vi "Update Status on Result.vi"(8 "error in (no error)":errorcluster, 10 "Result":T1, 11 "Execution UI V2 in":refnum<class "Execution UI V2.lvclass">) -> (0 "error out":errorcluster, 3 "Execution UI V2 out":refnum<class "Execution UI V2.lvclass">)   [LabVIEW 2020, in "Execution UI V2.lvclass"]
uses:
  Execution UI V2.lvclass
  Result/Result.ctl
  Result/Status.ctl
  Result/Type.ctl
  Result/Result.lvlib
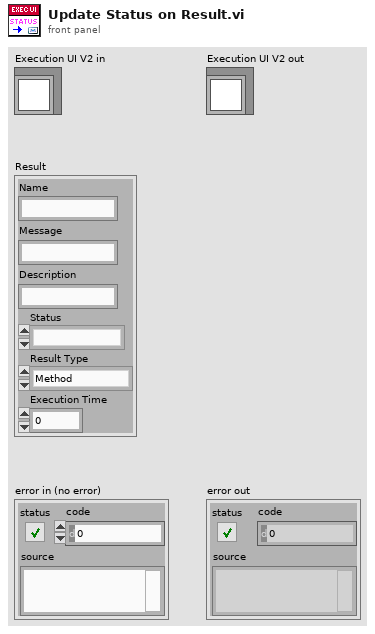
[diagram p1: front panel]
types:
  T1 = typedef "Result.lvlib/Result.ctl" = cluster{"Name":string, "Message":string, "Description":string, "Status":T2, "Result Type":T3, "Execution Time":dbl}
  T2 = typedef "Result.lvlib/Status.ctl" = enum16{"", "Passed", "Failed", "Error", "Skipped", "Setup Error", "Broken", "Teardown Error"}
  T3 = typedef "Result.lvlib/Type.ctl" = enum16{"Method", "Case", "Suite", "Pass", "Fail", "Skip", "Pass if", "Fail if", "Pass if Error", "Fail if Error", "Pass if Equal", "Fail if Equal"}
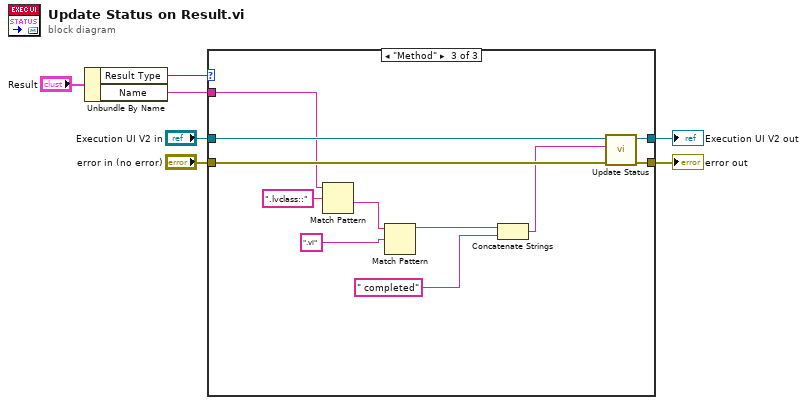
[diagram p0: block diagram]
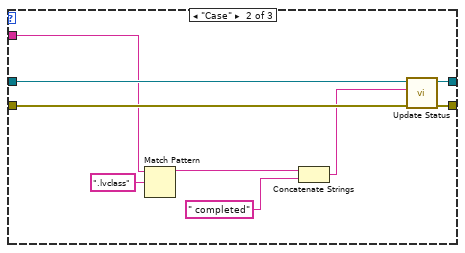
[diagram p3: hidden frame]
diagram:
  n1 = Unbundle By Name("Result") -> ("Result Type"=w7:T3, "Name"=w1:string)
  n2 = case shown="\"Method\"" w7 {
    tunnel: "Execution UI V2 in" -> [w9 w18 w29]
    tunnel: [w9 w17 w28] -> w3
    tunnel: "error in (no error)" -> [w8 w16 w27]
    tunnel: [w8 w15 w26] -> w5
    tunnel: w1 -> [_ w13 w21]
    frame Default {
    }
    frame "Case" {
      n3 = Match Pattern(string=w13, regular expression=".lvclass") -> (before substring=w11:string)  [unwired: 1 in, 3 out]
      n4 = Concatenate Strings(w11, " completed" ("Status")) -> (w10:string)
      n5 = call "Update Status.vi"("error in (no error)"=w16, "Status"=w10, "Execution UI In"=w18) -> ("error out"=w15:errorcluster, "Execution UI Out"=w17:refnum<class "Execution UI V2.lvclass">)  [unwired: 7 in]
    }
    frame "Method" {
      n6 = Match Pattern(string=w21, regular expression=".lvclass::") -> (after substring=w19:string)  [unwired: 1 in, 3 out]
      n7 = Match Pattern(string=w19, regular expression=".vi") -> (before substring=w23:string)  [unwired: 1 in, 3 out]
      n8 = Concatenate Strings(w23, " completed" ("Status")) -> (w22:string)
      n9 = call "Update Status.vi"("error in (no error)"=w27, "Status"=w22, "Execution UI In"=w29) -> ("error out"=w26:errorcluster, "Execution UI Out"=w28:refnum<class "Execution UI V2.lvclass">)  [unwired: 7 in]
    }
  }
  "error out" <- w5
  "Execution UI V2 out" <- w3
